vi "GetType.vi"(8 "error in (no error)":errorcluster, 11 "Initiate Acquisition Msg":refnum<class "Initiate Acquisition Msg.lvclass">) -> (0 "error out":errorcluster, 2 "Data Sample":variant, 3 "Initiate Acquisition Msg":refnum<class "Initiate Acquisition Msg.lvclass">)   [LabVIEW 2016, in "CS++Scope.lvlib" / "Initiate Acquisition Msg.lvclass"]
doc: "This VI delivers a sample of the data type format the message expects."
uses:
  Initiate Acquisition Msg.lvclass
  Initiate Acquisition Msg.lvclass/Initiate Acquisition Msg.ctl
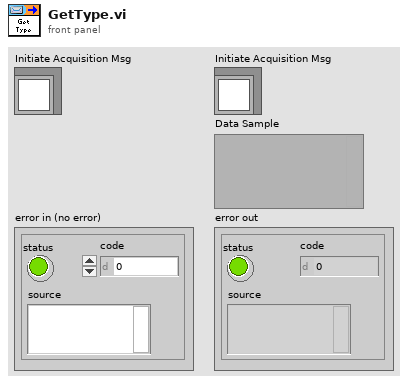
[diagram p1: front panel]
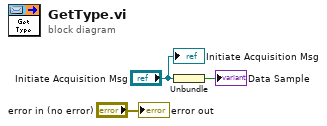
[diagram p0: block diagram]
diagram:
  n1 = Unbundle("Initiate Acquisition Msg") -> (→"Data Sample":bool)
  "error out" <- "error in (no error)"
  "Initiate Acquisition Msg" <- "Initiate Acquisition Msg"
